vi "BuildQueueName.vi"(11 "VI in":refnum<vi>) -> (0 "error out":errorcluster, 3 "Queue out":refnum<queue>)   [LabVIEW 2022 SP3]
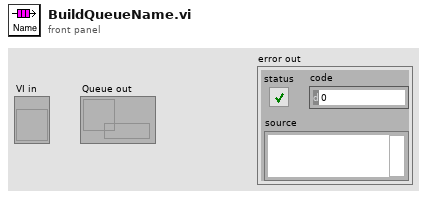
[diagram p1: front panel]
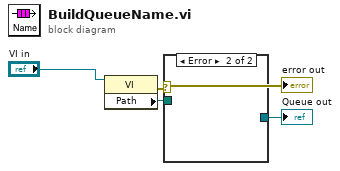
[diagram p0: block diagram]
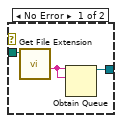
[diagram p2: hidden frame]
diagram:
  n1 = property class="VI"(reference="VI in") -> (error out=w1:errorcluster, "Path"=w3:path)  [unwired: 1 in, 1 out]
  "error out" <- w1
  n2 = case shown="Error" w1 {
    tunnel: [w7 _] -> w4
    tunnel: w3 -> [w5 _]
    frame No Error {
      n3 = call <vilib>:"Get File Extension.vi"("file"=w5) -> ("filename without extension"=w6:string)  [unwired: 6 in, 4 out]
      n4 = Obtain Queue(name (unnamed)=w6, element data type=w6) -> (queue out=w7:refnum<queue>)  [unwired: 3 in, 2 out]
    }
    frame Error {
    }
  }
  "Queue out" <- w4
